vi "串口.vi"() -> ()   [LabVIEW 2018]
uses:
  <vilib>/Instr/_visa.llb/VISA Configure Serial Port (Instr).vi
panel:
  in  "VISA resource name":refnum<visa-resource-name> caption="串口"
  in  "停止":bool
  out "接收命令":string
  in  "发送命令":string
  in  "写":bool
  in  "读":bool
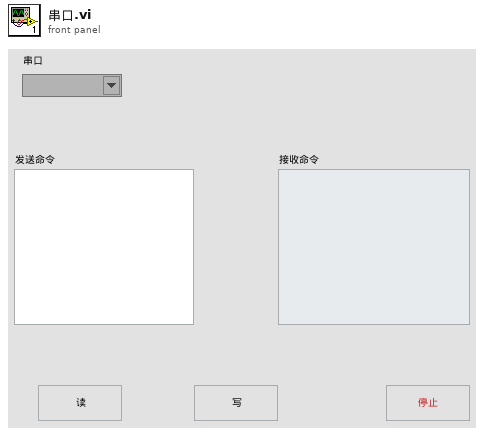
[diagram p1: front panel]
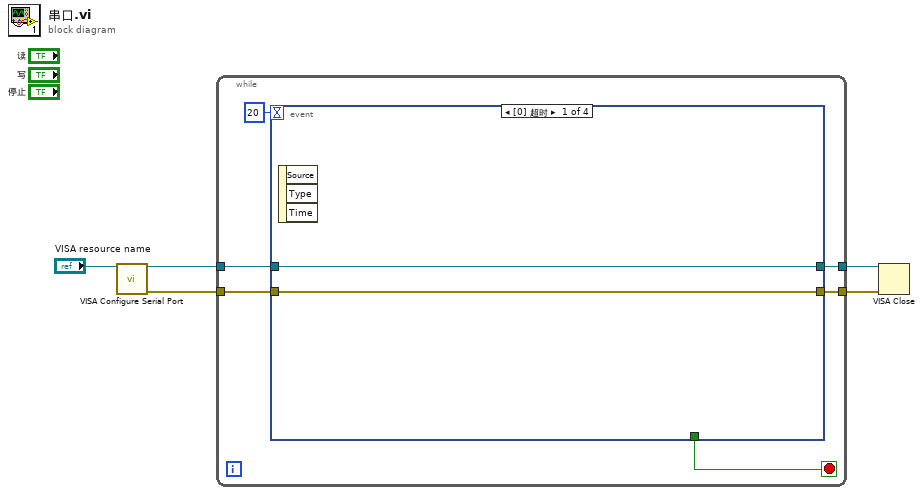
[diagram p0: block diagram]
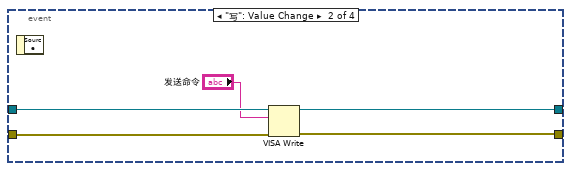
[diagram p2: hidden frame]
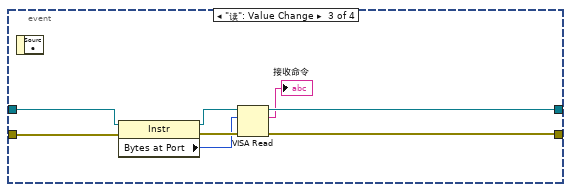
[diagram p3: hidden frame]
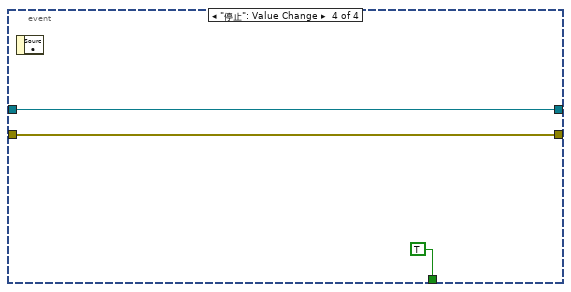
[diagram p4: hidden frame]
diagram:
  n1 = call-poly "VISA Configure Serial Port"("VISA resource name"="VISA resource name") -> ("VISA resource name out"=w4:refnum<visa-resource-name>, "error out"=w5:errorcluster)  [unwired: 13 in]
  n2 = while {
    tunnel: w5 -> [w11]
    tunnel: w4 -> [w9]
    tunnel: [w8] -> w3
    tunnel: [w7] -> w2
    stop <- w6 stop-if-true
    n3 = event shown="[0] 超时" {
      selector: _ -> [_ _ _ _]
      dyn-events: _ -> [_ _ _ _]
      timeout: 20 -> [_ _ _ _]
      tunnel: w11 -> [w12 w16 w23 w27]
      tunnel: w9 -> [w13 w18 w24 w28]
      tunnel: [w13 w17 w26 w28] -> w8
      tunnel: [w12 w15 w25 w27] -> w7
      tunnel: [_ _ _ TRUE] -> w6
      event Timeout {
        n4 = event-data() -> ()  [unwired: 1 in, 3 out]
      }
      event "写": Value Change {
        n5 = event-data() -> ()  [unwired: 1 in, 1 out]
        n6 = VISA Write(VISA resource name=w18, write buffer="发送命令", error in (no error)=w16) -> (VISA resource name out=w17:refnum<visa-resource-name>, error out=w15:errorcluster)  [unwired: 1 out]
      }
      event "读": Value Change {
        n7 = event-data() -> ()  [unwired: 1 in, 1 out]
        n8 = property class="Instr"(reference=w24, error in=w23) -> (reference out=w22:refnum<visa-resource-name>, error out=w21:errorcluster, "Bytes at Port"=w20:u32)
        n9 = VISA Read(VISA resource name=w22, byte count=w20, error in (no error)=w21) -> (VISA resource name out=w26:refnum<visa-resource-name>, read buffer=→"接收命令":string, error out=w25:errorcluster)  [unwired: 1 out]
      }
      event "停止": Value Change {
        n10 = event-data() -> ()  [unwired: 1 in, 1 out]
      }
    }
  }
  n11 = VISA Close(VISA resource name=w3, error in (no error)=w2) -> ()  [unwired: 1 out]
